vi "Agilent3446X_Measure.vi"(8 "error in":errorcluster caption="错误输入", 11 "MyIndex":u8) -> (0 "error out":errorcluster caption="错误输出", 3 "Value":dbl)   [LabVIEW 2015]
uses:
  Agilent 3446X Series/Public/Data/Read (Single Point)1.vi
  Agilent 3446X Series/Agilent 3446X Series1.lvlib
panel:
  in  "单位":enum16{"没单位", "u级", "m级"}(ring)
  out "VISA resource out":refnum<visa-resource-name>
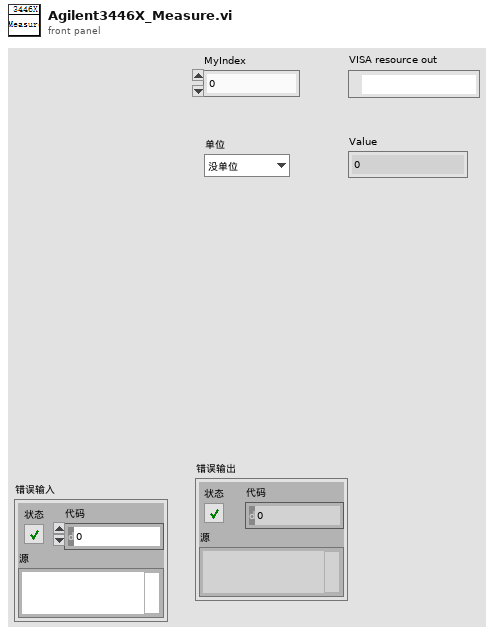
[diagram p1: front panel]
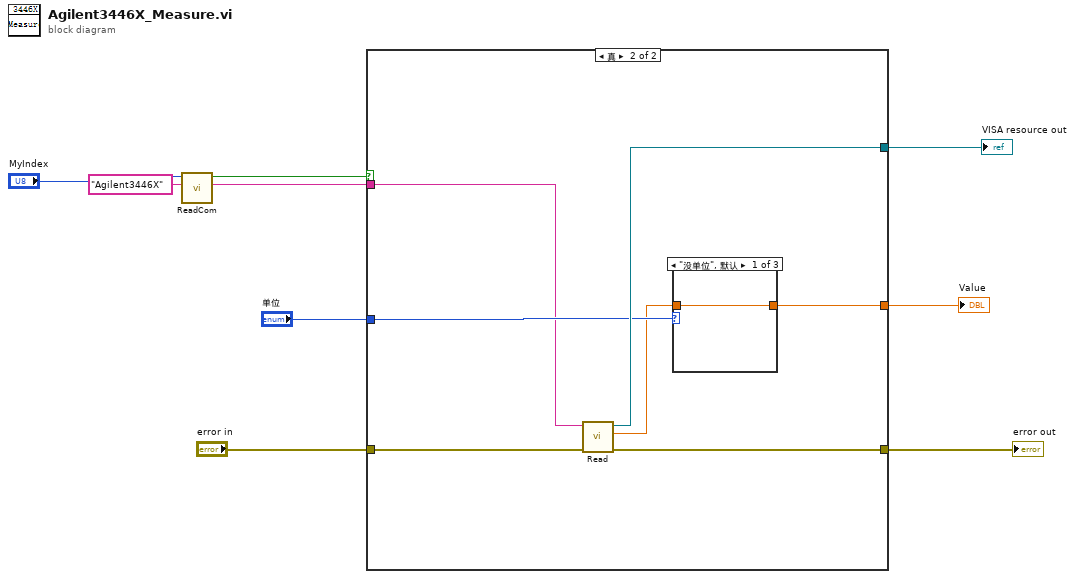
[diagram p0: block diagram]
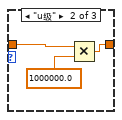
[diagram p3: hidden frame]
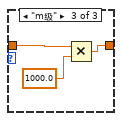
[diagram p4: hidden frame]
diagram:
  n1 = call "ReadCom.vi"("仪器名称"="Agilent3446X", "MyIndex"="MyIndex") -> ("COM"=w3:string, "OK?"=w4:bool)  [unwired: 7 in, 1 out]
  n2 = case shown="真" w4 {
    tunnel: [w10 w17] -> w9
    tunnel: [_ w16] -> w8
    tunnel: "单位" -> [_ w15]
    tunnel: w3 -> [_ w13]
    tunnel: "error in" -> [w10 w12]
    tunnel: [_ w11] -> w1
    frame False {
    }
    frame True {
      n3 = call-poly "Read.vi"("error in (no error)"=w12, "VISA resource name"=w13) -> ("error out"=w17:errorcluster, "Measurement"=w14:dbl, "VISA resource name out"=w16:refnum<visa-resource-name>)  [unwired: 7 out]
      n4 = case shown="\"没单位\", 默认" w15 {
        tunnel: w14 -> [w18 w21 w24]
        tunnel: [w18 w19 w22] -> w11
        frame "没单位", Default {
        }
        frame "u级" {
          n5 = Multiply(x=w21, y=1000000.0) -> (x*y=w19:dbl)
        }
        frame "m级" {
          n6 = Multiply(x=w24, y=1000.0) -> (x*y=w22:dbl)
        }
      }
    }
  }
  "error out" <- w9
  "VISA resource out" <- w8
  "Value" <- w1
